vi "Orca Flash Wait Ready.vi"(0 "Notifier Name":string, 11 "Error In":errorcluster) -> (4 "Notifier Name Out":string, 8 "Ready?":bool, 15 "Error Out":errorcluster)   [LabVIEW 2025]
uses:
  Orca Flash Controls/Orca Flash Notifier Element.ctl
  Orca Flash Controls/Orca Flash Actions.ctl
  Orca Flash Controls/Orca Flash Parameters.ctl
  Orca Flash Controls/Orca Flash Parameter List.ctl
  Orca Flash Controls/Orca Flash ROI.ctl
  <vilib>/vision/Image Controls.llb/IMAQ Image.ctl
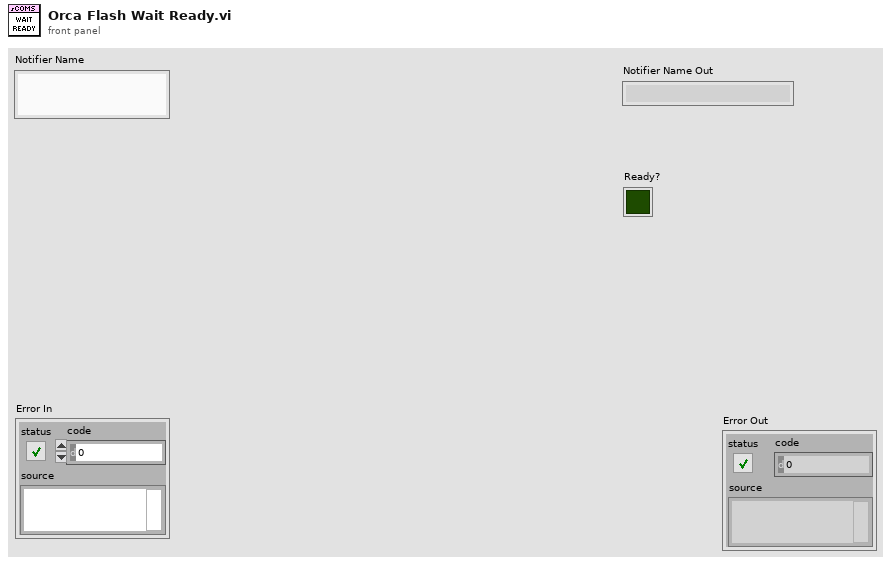
[diagram p1: front panel]
types:
  T1 = typedef "Orca Flash Notifier Element.ctl" = cluster{"Camera Actions":T2, "Received?":bool, "Running?":bool, "sCMOS Parameter":T3, "sCMOS ROI":T5, "Save Path":path, "# of frames":u32, "Image Ref":T6}
  T2 = typedef "Orca Flash Actions.ctl" = enum16{"Idle", "Preview", "Record", "Record Settings", "Set Param", "Get Param", "Set ROI", "Get ROI", "Trigger Source", "Trigger Type", "Progessive Mode", "Area Mode", "Status", "Quit"}
  T3 = typedef "Orca Flash Parameters.ctl" = cluster{"Value":dbl, "Parameter":T4}
  T4 = typedef "Orca Flash Parameter List.ctl" = u32
  T5 = typedef "Orca Flash ROI.ctl" = cluster{"H Offset":i32, "V Offset":i32, "H Width":i32, "V Width":i32}
  T6 = typedef "IMAQ Image.ctl" = refnum<image>
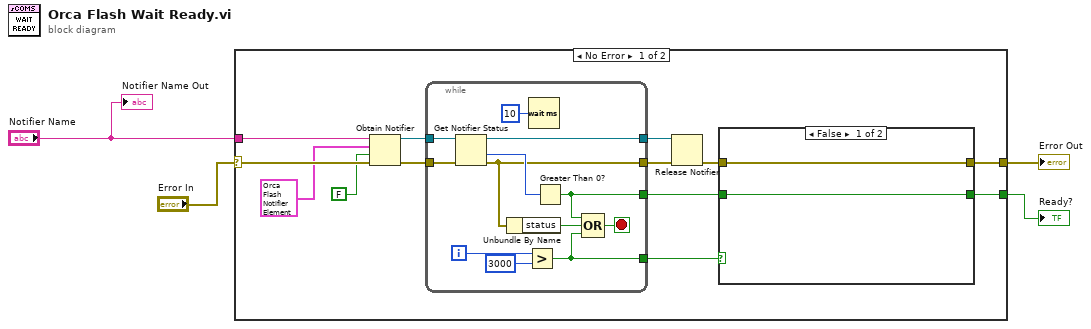
[diagram p0: block diagram]
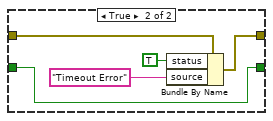
[diagram p2: hidden frame]
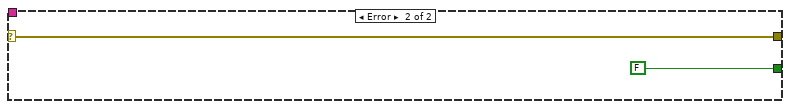
[diagram p3: hidden frame]
diagram:
  n1 = case shown="No Error" "Error In" {
    selector: "Error In" -> [w16 w38]
    tunnel: "Notifier Name" -> [w17 _]
    tunnel: [w15 FALSE] -> w3
    tunnel: [w14 w38] -> w2
    frame No Error {
      n2 = Obtain Notifier(name (unnamed)=w17, notification data type=T1 {"Camera Actions"=enum."Idle", "Received?"=FALSE, "Running?"=FALSE, "sCMOS Parameter"={"Value"=0.0, "Parameter"=4212128}, "sCMOS ROI"={"H Offset"=0, "V Offset"=0, "H Width"=0, "V Width"=0}, "Save Path"=path "", "# of frames"=0, "Image Ref"=refnum} ("Camera Cluster"), create if not found? (T)=FALSE, error in (no error)=w16) -> (notifier out=w12:refnum<notifier>, error out=w11:errorcluster)  [unwired: 1 out]
      n3 = while {
        tunnel: w12 -> [w36]
        tunnel: w11 -> [w35]
        tunnel: [w33] -> w6
        tunnel: [w27] -> w9
        tunnel: [w26] -> w10
        tunnel: [w25] -> w7
        i -> [w31]
        stop <- w28 stop-if-true
        n4 = Get Notifier Status(notifier=w36, error in (no error)=w35) -> (notifier out=w25:refnum<notifier>, # waiting=w34:i32, error out=w33:errorcluster)  [unwired: 2 out]
        n5 = Unbundle By Name(w33) -> ("status"=w29:bool)
        n6 = Greater?(x=w31, y=3000) -> (0:w26:bool)
        n7 = Wait (ms)(milliseconds to wait=u32 10) -> ()  [unwired: 1 out]
        n8 = Greater Than 0?(x=w34) -> (x > 0?=w27:bool)
        n9 = Compound Arithmetic op=OR(w27, w29, w26) -> (w28:bool)
      }
      n10 = Release Notifier(notifier=w7, error in (no error)=w6) -> (error out=w5:errorcluster)  [unwired: 1 in, 2 out]
      n11 = case shown="False" w10 {
        tunnel: w9 -> [w19 w20]
        tunnel: [w19 w20] -> w15
        tunnel: w5 -> [w18 w24]
        tunnel: [w18 w22] -> w14
        frame False {
        }
        frame True {
          n12 = Bundle By Name(cluster=w24, "status"=TRUE, "source"="Timeout Error") -> (w22:errorcluster)
        }
      }
    }
    frame Error {
    }
  }
  "Error Out" <- w2
  "Ready?" <- w3
  "Notifier Name Out" <- "Notifier Name"
